vi "GetDeviceInfoTDaqNDaqmx2.vi"() -> ()   [LabVIEW 2014]
uses:
  <resource>/objmgr/daqmx.rc
panel:
  in  "Driver":enum32{"NI-DAQmx", "Traditional NI-DAQ"}(tab)
  out "NI-DAQmx Device Names":string[](array[string])
  out "NI-DAQmx Devices":tag[](array[tag])
  # "Instructions:\n1) Select the appropriate tab based on which driver you want to use.\n2) Click the run button."
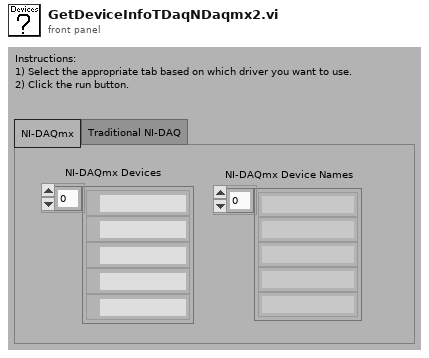
[diagram p1: front panel]
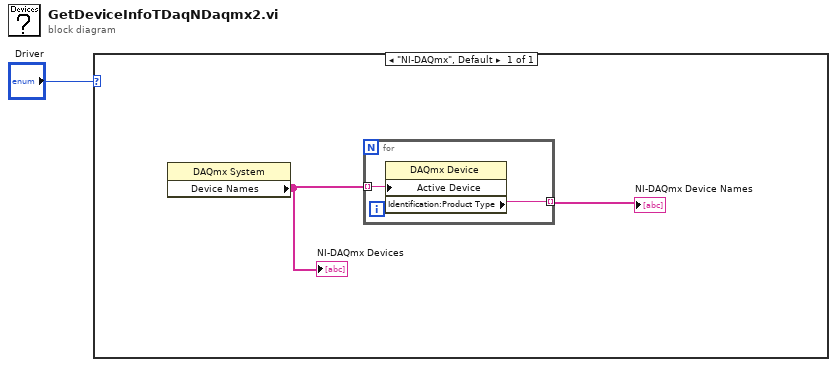
[diagram p0: block diagram]
diagram:
  n1 = case shown="\"NI-DAQmx\", Default" "Driver" {
    frame "NI-DAQmx", Default {
      n2 = property class="DAQmx System"() -> ("Device Names"=w3:tag[])  [unwired: 2 in, 2 out]
      "NI-DAQmx Devices" <- w3
      n3 = for {
        tunnel: w3 -> [w5] mode=indexing
        tunnel: [w4] -> w2 mode=indexing
        n4 = property class="DAQmx Device"("Active Device"=w5) -> ("Identification:Product Type"=w4:string)  [unwired: 2 in, 2 out]
      }
      "NI-DAQmx Device Names" <- w2
    }
  }
